vi "DHE_GetNbufs.vi"() -> (7 "DHE_Nbufs":u16)   [LabVIEW 2016]
uses:
  private/vis/DHE_GBLDriverVariables.vi
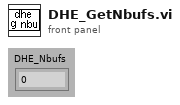
[diagram p1: front panel]
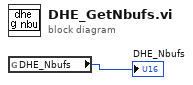
[diagram p0: block diagram]
diagram:
  n1 = global read "DHE_GBLDriverVariables.vi" "DHE_Nbufs"() -> (→"DHE_Nbufs":u16)
